vi "Excel___Create Certificate.vi"(0 "DataFilePath":path, 2 "Action to Perform":u16(ring) items=["", "Start Calibration", "Continue Calibration", "System Initialization", "System Closeout"], 5 "TemplatePath":path, 7 "Data":T3(array[cluster]), 9 "Tolerancing Bundle":T2(array[cluster]), 11 "Error In":errorcluster, 13 "All_Data":T1={"Environment Details"=[["TI Automotive"], ["Caro Test Center"], ["628 Columbia St."], ["Caro, MI 48723"], [""], [""], [""]], "Instrument Identification"=[], "Standards Used"=[], "Calibration Details"=[], "Machine Specifications:"=[], "Channel Descriptions:"=[], "Tracking"=[], "CalChannelsAsFound"=[], "CalChannelsCalibrate"=[], "CalChannelsVerify"=[], "Coefficients"=[], "CalDueDates"=[]}) -> (15 "Error Out":errorcluster)   [LabVIEW 2013]
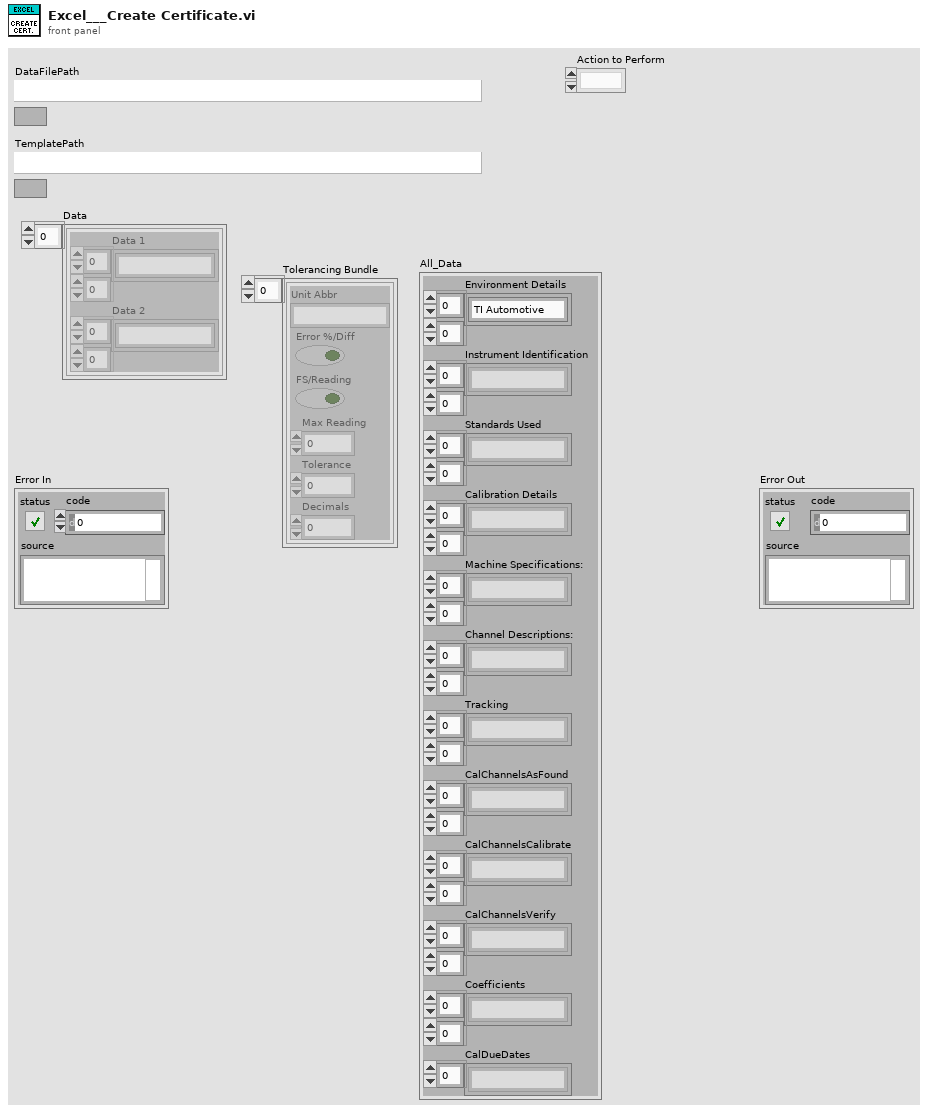
[diagram p1: front panel]
types:
  T1 = cluster{"Environment Details":string[][], "Instrument Identification":string[][], "Standards Used":string[][], "Calibration Details":string[][], "Machine Specifications:":string[][], "Channel Descriptions:":string[][], "Tracking":string[][], "CalChannelsAsFound":string[][], "CalChannelsCalibrate":string[][], "CalChannelsVerify":string[][], "Coefficients":string[][], "CalDueDates":string[]}
  T2 = cluster{"Unit Abbr":string, "Error %/Diff":bool, "FS/Reading":bool, "Max Reading":dbl, "Tolerance":dbl, "Decimals":i16}[]
  T3 = cluster{"Data 1":string[][], "Data 2":string[][]}[]
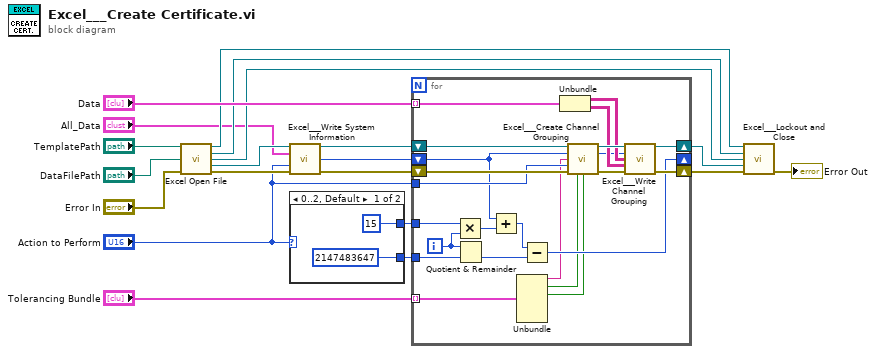
[diagram p0: block diagram]
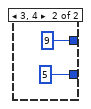
[diagram p2: hidden frame]
diagram:
  n1 = call "Excel Open File.vi"("TemplatePath"="TemplatePath", "DataFilePath"="DataFilePath", "Error In"="Error In") -> ("Excel Ref Out"=w8:refnum<k7>, "WorkbookS Ref Out"=w9:refnum<k7>, "Workbook Ref Out"=w10:refnum<k7>, "Sheets Ref Out"=w16:refnum<k7>, "Error Out"=w17:errorcluster)  [unwired: 8 in]
  n2 = call "Excel___Write System Information.vi"("Sheets Ref In"=w16, "All_Data"="All_Data", "Action to Perform"="Action to Perform", "Error In"=w17) -> ("Sheets Ref Out"=w15:refnum<k7>, "Starting Index"=w4:i32, "Error Out"=w14:errorcluster)  [unwired: 9 in]
  n3 = case shown="0..2, Default" "Action to Perform" {
    tunnel: [2147483647 ("y") 5 ("y")] -> w13
    tunnel: [15 ("x") 9 ("x")] -> w12
    frame 0..2, Default {
    }
    frame 3, 4 {
    }
  }
  n4 = for {
    shift-right: [w41] -> w7
    shift-left: w15 -> [w46]
    shift-right: [w43] -> w6
    shift-left: w14 -> [w45]
    shift-right: [w30] -> _
    shift-left: w4 -> [w32]
    tunnel: w12 -> [w39]
    tunnel: w13 -> [w38]
    tunnel: "Data" -> [w37] mode=indexing
    tunnel: "Action to Perform" -> [w34]
    tunnel: "Tolerancing Bundle" -> [w28] mode=indexing
    i -> [w40]
    n5 = Multiply(x=w39, y=w40) -> (x*y=w33:i32)
    n6 = Quotient & Remainder(x=w40, y=w38) -> (floor(x/y)=w29:i32)  [unwired: 1 out]
    n7 = Add(x=w32, y=w33) -> (x+y=w31:i32)
    n8 = Unbundle(w28) -> ("Unit Abbr"=w25:string, "Error %/Diff"=w27:bool, "FS/Reading"=w26:bool)  [unwired: 3 out]
    n9 = Subtract(x=w31, y=w29) -> (x-y=w30:i32)
    n10 = Unbundle(w37) -> ("Data 1"=w36:string[][], "Data 2"=w35:string[][])
    n11 = call "Excel___Create Channel Grouping.vi"("Sheets Ref In"=w46, "Starting Row"=w32, "Units String"=w25, "Action to Perform"=w34, "Error In"=w45, "Percent Error(F)"=w27, "FS(T)/Reading(F)"=w26) -> ("Sheets Ref Out"=w42:refnum<k7>, "Error Out"=w44:errorcluster)  [unwired: 7 in]
    n12 = call "Excel___Write Channel Grouping.vi"("Sheets Ref In"=w42, "Starting Row"=w32, "Data 1"=w36, "Data 2"=w35, "Error In"=w44) -> ("Sheets Ref Out"=w41:refnum<k7>, "Error Out"=w43:errorcluster)  [unwired: 9 in]
  }
  n13 = call "Excel___Lockout and Close.vi"("Excel Ref In"=w8, "WorkbookS Ref In"=w9, "Workbook Ref In"=w10, "Sheets Ref In"=w7, "Error In"=w6) -> ("Error Out"=→"Error Out":errorcluster)  [unwired: 10 in]
